vi "ISX3_Write_Data.vi"(4 "Data to Write":u8[](array[numeric]), 5 "FT_Handle":u32) -> (1 "Bytes Written":u32, 2 "FT_Handle":u32)   [LabVIEW 2012, in "Sciospec ISX3 Impedance Analyzer.lvlib"]
uses:
  Sciospec ISX3 Impedance Analyzer.lvlib
panel:
  # "FT_Handle to the USB interface"
  # "Bytes written to the interface.\nIf an error occurs while writing to interface \nthis number will differ from the length of \"Data To write\""
  # "Data to write to the interface"
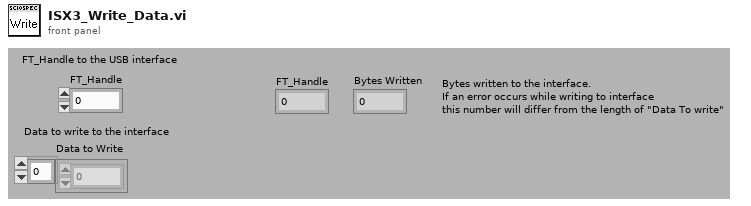
[diagram p1: front panel]
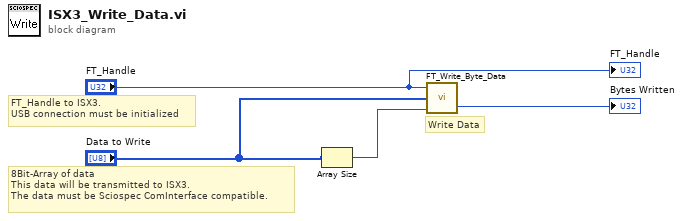
[diagram p0: block diagram]
diagram:
  # "Write Data"
  # "8Bit-Array of data\nThis data will be transmitted to ISX3.\nThe data must be Sciospec ComInterface compatible."
  # "FT_Handle to ISX3.\nUSB connection must be initialized"
  n1 = Array Size(array="Data to Write") -> (size(s)=w3:i32)
  n2 = call "FT_Write_Byte_Data.vi"("Bytes To Write"=w3, "Buffer"="Data to Write", "Handle"="FT_Handle") -> ("Bytes Written"=→"Bytes Written":u32)  [unwired: 1 out]
  "FT_Handle" <- "FT_Handle"
